vi "dfd_2-band Lattice Coefficients Optimization.vi"(8 "error in (no error)":errorcluster, 9 "roll-off":dbl=0.2, 11 "coef":dbl[](array[numeric])) -> (0 "error out":errorcluster, 3 "coef":dbl[](array[numeric]))   [LabVIEW 2017, in "NI_DigFilter_FilterBank.lvlib"]
doc: "This VI shows an example of using the Unconstrained Optimization VI. The VI uses the Extended Rosenbrock Function VI to create an objective function. The VI then passes this function to the Unconstrained Optimization VI."
uses:
  <vilib>/addons/Digital Filter Design/NI_DigFilter_FilterBank.lvlib
  <vilib>/gmath/NumericalOptimization/stopping criteria.ctl
  <vilib>/gmath/NumericalOptimization/Quasi Newton.vi
  <vilib>/gmath/NI_Gmath.lvlib
  <vilib>/addons/Digital Filter Design/NI_DigFilterLicensed.lvlib
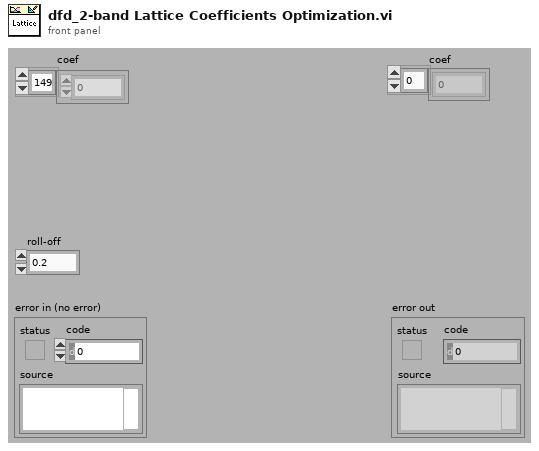
[diagram p1: front panel]
types:
  T1 = typedef "NI_Gmath.lvlib/stopping criteria.ctl" = cluster{"function tolerance":dbl, "parameter tolerance":dbl, "max iterations":i32, "max function calls":i32, "gradient tolerance":dbl, "max time (sec)":dbl}
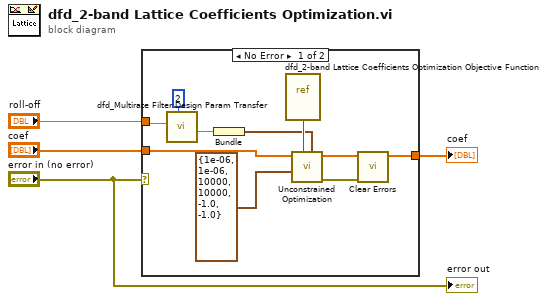
[diagram p0: block diagram]
diagram:
  n1 = case shown="No Error" "error in (no error)" {
    tunnel: "coef" -> [w11 _]
    tunnel: [w10 _] -> w1
    tunnel: "roll-off" -> [w6 _]
    frame No Error {
      n2 = call <vilib>:"dfd_Multirate Filter Design Param Transfer.vi"("multirate factor"=2, "roll off"=w6) -> ("fstop"=w5:dbl)  [unwired: 4 in, 5 out]
      n3 = Bundle("fstop"=w5) -> (w8:cluster{"fstop":dbl})  [unwired: 1 in]
      n4 = vi-ref <vilib>:"dfd_2-band Lattice Coefficients Optimization Objective Function.vi"() -> (w12:refnum<vi>)
      n5 = call-poly <vilib>:"Unconstrained Optimization.vi"("function data"=w8, "objective function"=w12, "stopping criteria"=T1 {"function tolerance"=1e-06, "parameter tolerance"=1e-06, "max iterations"=10000, "max function calls"=10000, "gradient tolerance"=-1.0, "max time (sec)"=-1.0}, "start"=w11) -> ("error out"=w9:errorcluster, "minimum"=w10:dbl[])  [unwired: 4 in, 2 out]
      n6 = call <vilib>:"Clear Errors.vi"("error in (no error)"=w9) -> ()  [unwired: 5 in, 2 out]
    }
    frame Error {
    }
  }
  "coef" <- w1
  "error out" <- "error in (no error)"
